vi "Measurement UI.vi"() -> ()   [LabVIEW 2021, in "audio_acMeasurement.lvlib"]
uses:
  audio_acMeasurement.lvlib
panel:
  in  "MeasGraphs":T1(tab)
  out "FreqDomainGraph":cluster{"x0":dbl, "dx":dbl, "magnitude":dbl[]}(graph) caption="AC"
  out "TimeDomainGraph":waveform(dbl)(graph) caption="AC"
  out "Channel":string
  out "Spectrum":dbl[](array[numeric])
  out "df":dbl
  out "f0":dbl
  out "Time domain":dbl[](array[numeric])
  out "dt":dbl
  out "THD+N":dbl
  out "THD":dbl
  out "SNR":dbl
  out "Calculated amplitude":dbl
  out "Calculated frequency":dbl
  out "SFDR":dbl
  out "Dynamic range":dbl
  out "Gain error":dbl
  in  "Analog source resource name":string
  out "MeasTable":string[][](table)
  in  "Channel name":string caption="CHANNEL NAME"
  in  "Channel":u32 caption="CHANNEL"
  in  "Data line":u16 caption="DATA LINE"
  out "Calculated sample rate":u32 caption="SAMPLE RATE" format="%#.6pHz"
  in  "Protocol capture resource name":string caption="RESOURCE NAME"
  in  "Protocol settings":string="Protocol settings"
  in  "Analog source":string="Analog source "
  in  "Full scale range":dbl=3.16 caption="FULL SCALE RANGE" format="%.3pV"
  in  "Measurement settings":string="Measurement settings"
  in  "MeasSettingsOptions":i32(listbox)=-1
  in  "MeasSettings":bool
  in  "Protocol":u16(ring) caption="PROTOCOL" items=["I2S"]
  in  "DSGResourceName":tag caption="RESOURCE NAME"
  in  "Weighting filter":T2(ring) caption="WEIGHTING FILTER"
  in  "Number of words":i32=19200 caption="NUMBER OF WORDS"
  in  "Clock rate":u32=12288000 caption="CLOCK RATE" format="%#.6pHz"
  in  "Band stop":dbl=20000.0 caption="BAND STOP" format="%#_6pHz"
  in  "Band start":dbl=20.0 caption="BAND START" format="%#_6pHz"
  in  "Amplitude":dbl=-1.0 caption="AMPLITUDE" format="%#_6pdB"
  in  "Frequency":dbl=1000.0 caption="FREQUENCY" format="%#_6pHz"
  in  "Sensitivity":dbl=0.34762 caption="SENSITIVITY" format="%.5fFS/Pa"
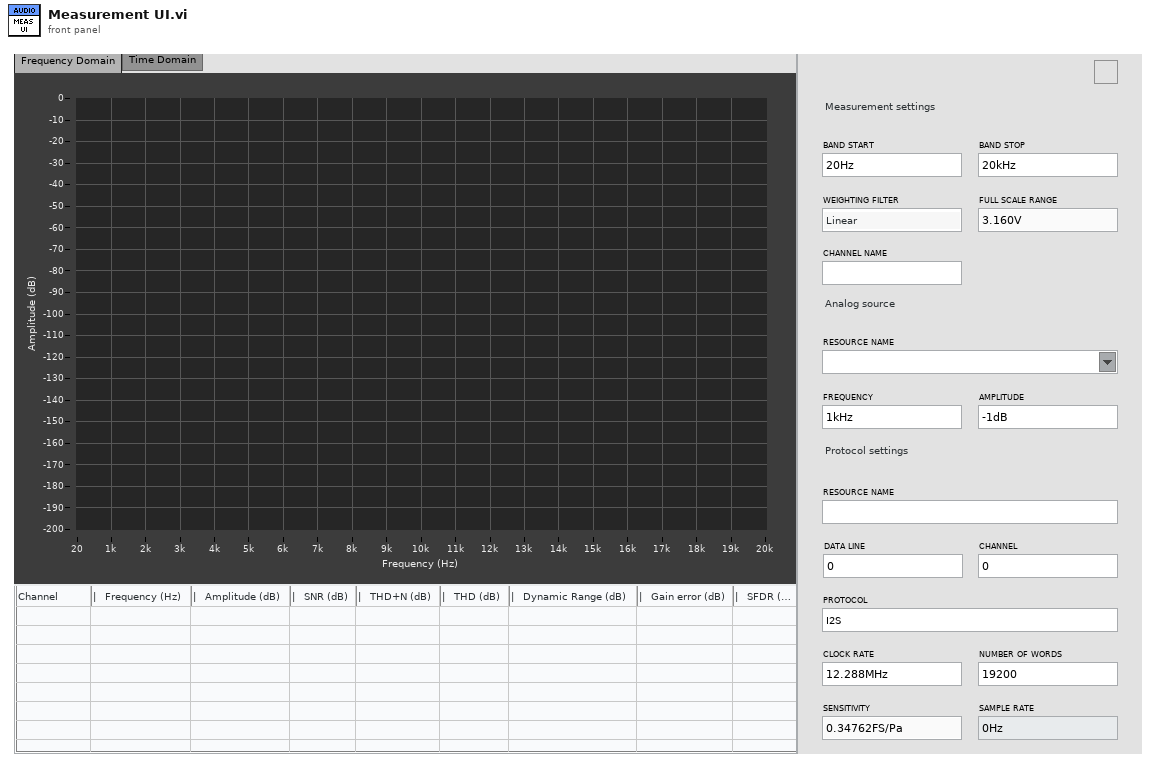
[diagram p1: front panel]
types:
  T1 = enum32{"Frequency Domain", "Time Domain", "Hidden Controls"}
  T2 = enum16{"Linear", "A-Weighting", "B-Weighting", "C-Weighting"}
  T3 = enum16{"open", "replace", "create", "open or create", "replace or create", "replace or create with confirmation"}
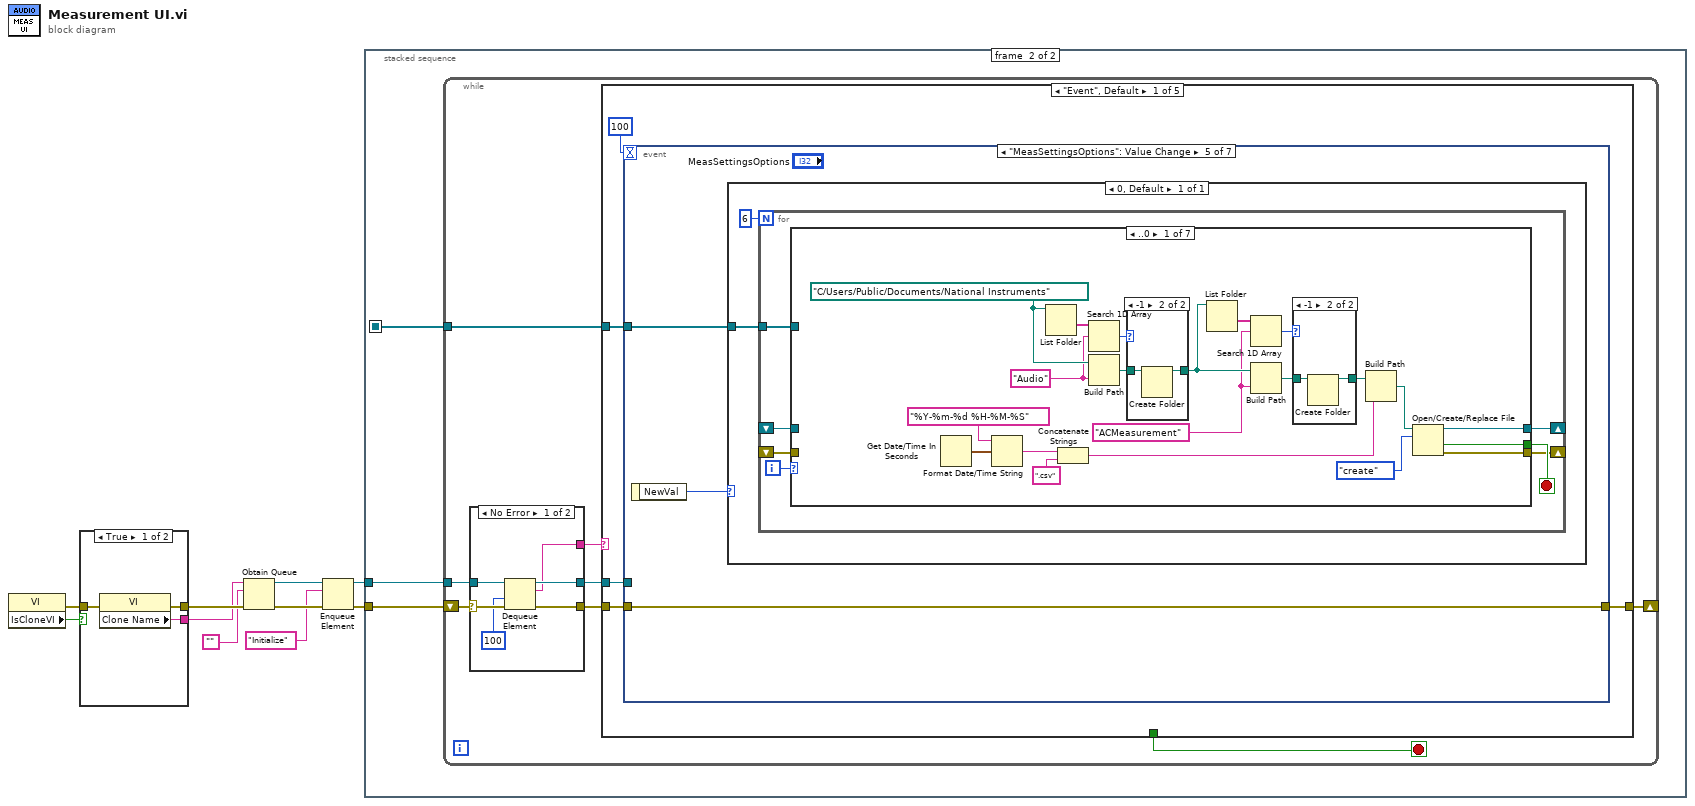
[diagram p0: block diagram]
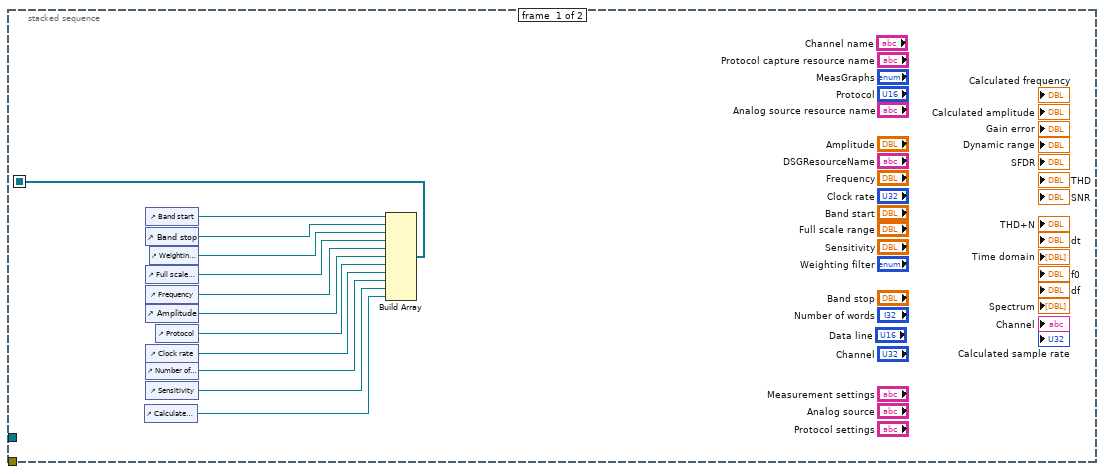
[diagram p2: hidden frame]
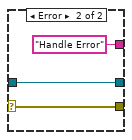
[diagram p3: hidden frame]
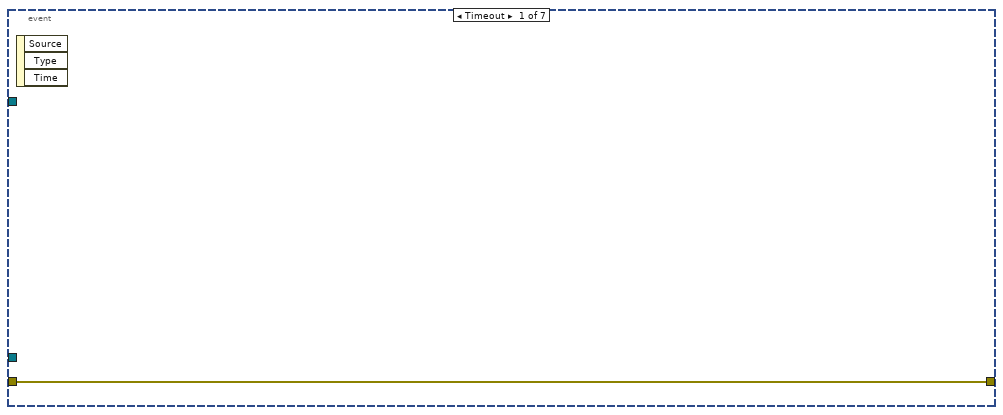
[diagram p4: hidden frame]
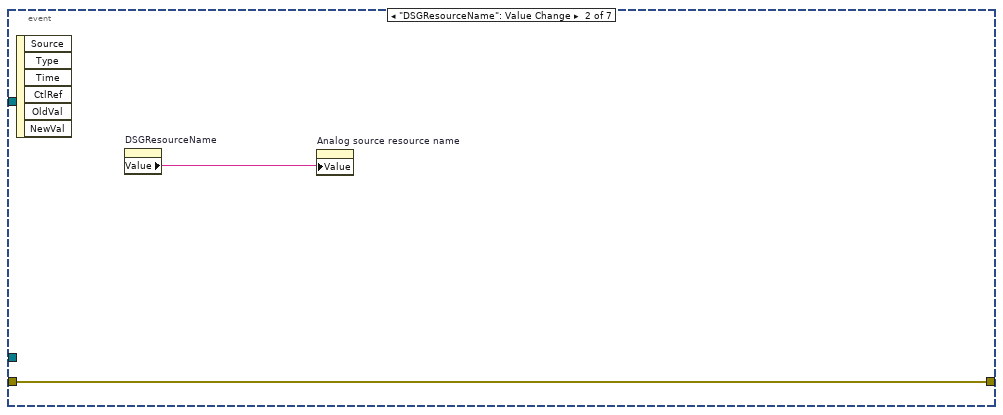
[diagram p5: hidden frame]
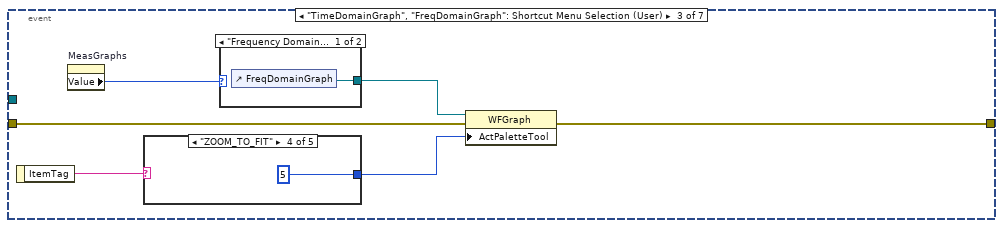
[diagram p6: hidden frame]
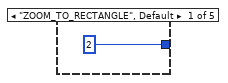
[diagram p7: hidden frame]
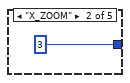
[diagram p8: hidden frame]
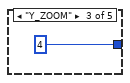
[diagram p9: hidden frame]
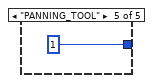
[diagram p10: hidden frame]
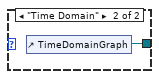
[diagram p11: hidden frame]
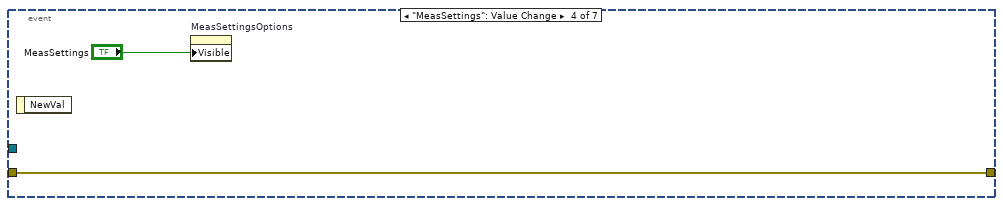
[diagram p12: hidden frame]
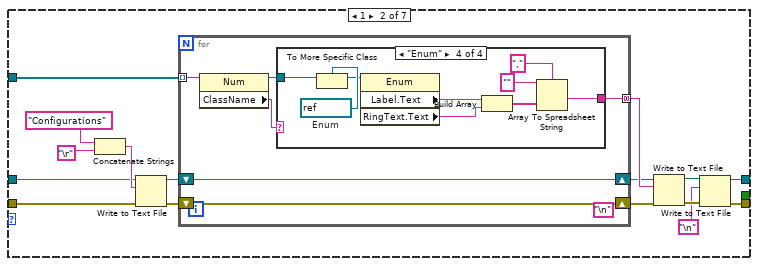
[diagram p15: hidden frame]
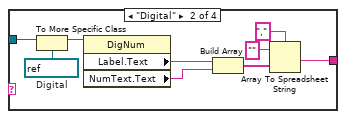
[diagram p17: hidden frame]
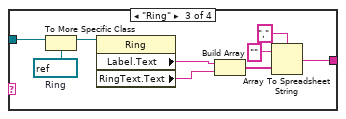
[diagram p18: hidden frame]
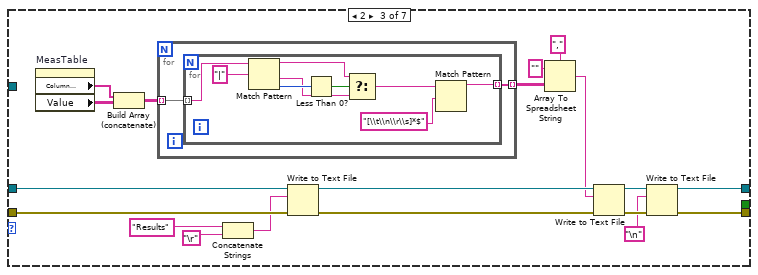
[diagram p19: hidden frame]
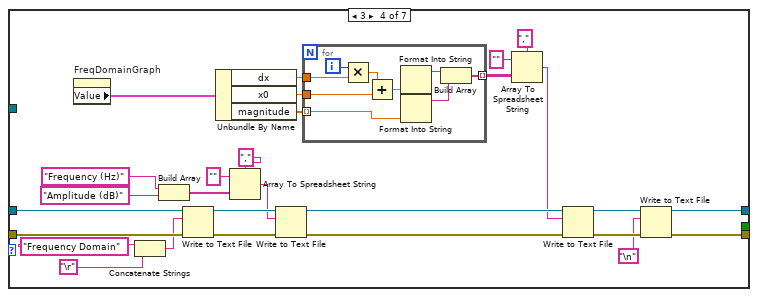
[diagram p20: hidden frame]
diagram:
  n1 = property class="VI"() -> (error out=w1:errorcluster, "IsCloneVI"=w2:bool)  [unwired: 2 in, 1 out]
  n2 = case shown="True" w2 {
    tunnel: [w13 w16] -> w10
    tunnel: [w12 w15] -> w9
    tunnel: w1 -> [w11 w14]
    frame True {
      n3 = property class="VI"(error in=w11) -> (error out=w13:errorcluster, "Clone Name"=w12:string)  [unwired: 1 in, 1 out]
    }
    frame False {
      n4 = property class="VI"(error in=w14) -> (error out=w16:errorcluster, "Name"=w15:string)  [unwired: 1 in, 1 out]
    }
  }
  n5 = Obtain Queue(name (unnamed)=w9, element data type="", error in (no error)=w10) -> (queue out=w6:refnum<queue>, error out=w8:errorcluster)  [unwired: 2 in, 1 out]
  n6 = Enqueue Element(queue=w6, element="Initialize", error in (no error)=w8) -> (queue out=w5:refnum<queue>, error out=w7:errorcluster)  [unwired: 1 in, 1 out]
  n7 = stacked-sequence {
    seq-local: [w25 _] -> [_ w29]
    tunnel: w7 -> [_ w31]
    tunnel: w5 -> [_ w30]
    frame #0 {
      n8 = control-ref of="Calculated sample rate"() -> (w17:refnum<vi>)
      n9 = control-ref of="Band start"() -> (w28:refnum<vi>)
      n10 = control-ref of="Band stop"() -> (w27:refnum<vi>)
      n11 = control-ref of="Full scale range"() -> (w24:refnum<vi>)
      n12 = control-ref of="Frequency"() -> (w21:refnum<vi>)
      n13 = control-ref of="Amplitude"() -> (w20:refnum<vi>)
      n14 = control-ref of="Clock rate"() -> (w23:refnum<vi>)
      n15 = control-ref of="Number of words"() -> (w19:refnum<vi>)
      n16 = control-ref of="Sensitivity"() -> (w18:refnum<vi>)
      n17 = control-ref of="Weighting filter"() -> (w26:refnum<vi>)
      n18 = control-ref of="Protocol"() -> (w22:refnum<vi>)
      n19 = Build Array(w28, w27, w26, w24, w21, w20, w22, w23, w19, w18, w17) -> (w25:refnum<vi>[])
    }
    frame #1 {
      n20 = while {
        shift-right: [w34] -> _
        shift-left: w31 -> [w39]
        tunnel: w30 -> [w37]
        tunnel: w29 -> [w32]
        stop <- w33 stop-if-true
        n21 = case shown="No Error" w39 {
          selector: w39 -> [w45 w48]
          tunnel: [w44 w48] -> w38
          tunnel: w37 -> [w43 w47]
          tunnel: [w42 w47] -> w36
          tunnel: [w41 "Handle Error"] -> w35
          frame No Error {
            n22 = Dequeue Element(queue=w43, timeout in ms (-1)=100, error in (no error)=w45) -> (queue out=w42:refnum<queue>, element=w41:string, error out=w44:errorcluster)  [unwired: 1 out]
          }
          frame Error {
          }
        }
        n23 = case shown="\"Event\", Default" w35 {
          tunnel: w38 -> [w52 w280 w318 w333 w334]
          tunnel: w36 -> [w50 _ _ w331 _]
          tunnel: [w53 w280 w318 w328 w334] -> w34
          tunnel: [_ _ _ TRUE _] -> w33
          tunnel: w32 -> [w49 _ _ _ _]
          frame "Event", Default {
            n24 = event shown="[4] \"MeasSettingsOptions\": Value Change" {
              selector: _ -> [_ _ _ _ _ _ _]
              dyn-events: _ -> [_ _ _ _ _ _ _]
              timeout: 100 -> [_ _ _ _ _ _ _]
              tunnel: [w54 w55 w59 _ w74 w266 w271] -> w53
              tunnel: w52 -> [w54 w55 w58 w70 w74 w266 w272]
              tunnel: w50 -> [_ _ _ _ _ _ w270]
              tunnel: [_ _ _ w70 _ _ _] -> _
              tunnel: w49 -> [_ _ _ _ w72 _ _]
              event Timeout {
                n25 = event-data() -> ()  [unwired: 1 in, 3 out]
              }
              event "DSGResourceName": Value Change {
                n26 = event-data() -> ()  [unwired: 1 in, 6 out]
                n27 = property on="DSGResourceName" class="DAQmxName"() -> ("Value"=w56:string)  [unwired: 2 in, 2 out]
                n28 = property on="Analog source resource name" class="Str"("Value"=w56) -> ()  [unwired: 2 in, 2 out]
              }
              event "TimeDomainGraph", "FreqDomainGraph": Shortcut Menu Selection (User) {
                n29 = event-data() -> ("ItemTag"=w61:string)  [unwired: 1 in]
                n30 = property on="MeasGraphs" class="TabCtl (strict)"() -> ("Value"=w62:T1)  [unwired: 2 in, 2 out]
                n31 = case shown="\"ZOOM_TO_FIT\"" w61 {
                  tunnel: [2 3 4 5 1] -> w57
                  frame "ZOOM_TO_RECTANGLE", Default {
                  }
                  frame "X_ZOOM" {
                  }
                  frame "Y_ZOOM" {
                  }
                  frame "ZOOM_TO_FIT" {
                  }
                  frame "PANNING_TOOL" {
                  }
                }
                n32 = case shown="\"Frequency Domain\", Default" w62 {
                  tunnel: [w68 w69] -> w60
                  frame "Frequency Domain", Default {
                    n33 = control-ref of="FreqDomainGraph"() -> (w68:refnum<vi>)
                  }
                  frame "Time Domain" {
                    n34 = control-ref of="TimeDomainGraph"() -> (w69:refnum<vi>)
                  }
                }
                n35 = property class="WFGraph"(reference=w60, error in=w58, "ActPaletteTool"=w57) -> (error out=w59:errorcluster)  [unwired: 1 out]
              }
              event "MeasSettings": Value Change {
                n36 = event-data() -> ()  [unwired: 1 in, 1 out]
                n37 = property on="MeasSettingsOptions" class="LstBox (strict)"("Visible"="MeasSettings") -> ()  [unwired: 2 in, 2 out]
              }
              event "MeasSettingsOptions": Value Change {
                n38 = event-data() -> ("NewVal"=w73:i32)  [unwired: 1 in]
                n39 = case shown="0, Default" w73 {
                  tunnel: w72 -> [w75]
                  frame 0, Default {
                    n40 = for {
                      N: 6 -> [_]
                      shift-right: [w81] -> _
                      shift-left: _ -> [w80]
                      shift-right: [w79] -> _
                      shift-left: _ -> [w78]
                      tunnel: w75 -> [w77]
                      i -> [w83]
                      stop <- w82 stop-if-true
                      n41 = case shown="..0" w83 {
                        tunnel: [w97 _ _ _ _ _ _] -> w82
                        tunnel: [w103 w123 w167 w194 w235 refnum<file> refnum ("refnum out") w265] -> w81
                        tunnel: w80 -> [_ w120 w178 w217 w236 w263 w265]
                        tunnel: [w96 w122 w166 w192 w234 w261 w264] -> w79
                        tunnel: w78 -> [_ w118 w177 w216 w237 w260 w264]
                        tunnel: w77 -> [_ w121 _ _ _ _ _]
                        frame ..0 {
                          w92 = "ACMeasurement" ("prompt")
                          w99 = "Audio" ("prompt")
                          w102 = path "C:/Users/Public/Documents/National Instruments" ("base path")
                          n42 = Get Date/Time In Seconds() -> (seconds since 1Jan1904=w89:timestamp)
                          n43 = Format Date/Time String(time format string (%c)="%Y-%m-%d %H-%M-%S", seconds (now)=w89) -> (date/time string=w88:string)  [unwired: 1 in]
                          n44 = List Folder(path=w102) -> (folder names=w100:string[])  [unwired: 3 in, 3 out]
                          n45 = Concatenate Strings(w88, ".csv" ("string")) -> (w85:string)
                          n46 = Search 1D Array(1D array=w100, element=w99) -> (index of element=w98:i32)  [unwired: 1 in]
                          n47 = Build Path(base path=w102, name or relative path=w99) -> (appended path=w101:path)
                          n48 = case shown="-1" w98 {
                            tunnel: w101 -> [w108 w110]
                            tunnel: [w108 w109] -> w93
                            frame Default {
                            }
                            frame -1 {
                              n49 = Create Folder(path (use dialog)=w110) -> (created path=w109:path)  [unwired: 2 in, 2 out]
                            }
                          }
                          n50 = List Folder(path=w93) -> (folder names=w95:string[])  [unwired: 3 in, 3 out]
                          n51 = Search 1D Array(1D array=w95, element=w92) -> (index of element=w94:i32)  [unwired: 1 in]
                          n52 = Build Path(base path=w93, name or relative path=w92) -> (appended path=w91:path)
                          n53 = case shown="-1" w94 {
                            tunnel: w91 -> [w105 w107]
                            tunnel: [w105 w106] -> w86
                            frame Default {
                            }
                            frame -1 {
                              n54 = Create Folder(path (use dialog)=w107) -> (created path=w106:path)  [unwired: 2 in, 2 out]
                            }
                          }
                          n55 = Build Path(base path=w86, name or relative path=w85) -> (appended path=w84:path)
                          n56 = Open/Create/Replace File(file path (use dialog)=w84, operation (0:open)=T3."create") -> (refnum out=w103:refnum<file>, cancelled=w97:bool, error out=w96:errorcluster)  [unwired: 4 in]
                        }
                        frame 1 {
                          (unwired) "\n"
                          n57 = Concatenate Strings("Configurations" ("format string"), "\r") -> (w124:string)
                          n58 = Write to Text File(file (use dialog)=w120, text=w124, error in=w118) -> (refnum out=w117:refnum<file>, error out=w119:errorcluster)  [unwired: 1 in, 1 out]
                          n59 = for {
                            tunnel: w121 -> [w128] mode=indexing
                            shift-right: [w132] -> w115
                            shift-left: w117 -> [w132]
                            shift-right: [w131] -> w114
                            shift-left: w119 -> [w131]
                            tunnel: [w130] -> w116 mode=concatenating
                            n60 = property class="Num"(reference=w128) -> (reference out=w129:refnum<vi>, "ClassName"=w127:string)  [unwired: 1 in, 1 out]
                            n61 = case shown="\"Enum\"" w127 {
                              tunnel: [_ w136 w146 w155] -> w130
                              tunnel: w129 -> [_ w134 w144 w159]
                              frame Default {
                              }
                              frame "Digital" {
                                w133 = refnum<vi> refnum  # Digital
                                n62 = To More Specific Class(target class=w133, reference=w134) -> (specific class reference=w135:refnum<vi>)  [unwired: 1 in, 1 out]
                                n63 = property class="DigNum"(reference=w135) -> ("Label.Text"=w141:string, "NumText.Text"=w140:string)  [unwired: 1 in, 2 out]
                                n64 = Build Array(w141, w140) -> (w137:string[])
                                n65 = Array To Spreadsheet String(delimiter (Tab)=",", array=w137, 3:"" ("format string")) -> (spreadsheet string=w136:string)
                              }
                              frame "Ring" {
                                w143 = refnum<vi> refnum  # Ring
                                n66 = To More Specific Class(target class=w143, reference=w144) -> (specific class reference=w145:refnum<vi>)  [unwired: 1 in, 1 out]
                                n67 = property class="Ring"(reference=w145) -> ("Label.Text"=w142:string, "RingText.Text"=w150:string)  [unwired: 1 in, 2 out]
                                n68 = Build Array(w142, w150) -> (w147:string[])
                                n69 = Array To Spreadsheet String(delimiter (Tab)=",", array=w147, 3:"" ("format string")) -> (spreadsheet string=w146:string)
                              }
                              frame "Enum" {
                                w158 = refnum<vi> refnum  # Enum
                                n70 = To More Specific Class(target class=w158, reference=w159) -> (specific class reference=w154:refnum<vi>)  [unwired: 1 in, 1 out]
                                n71 = property class="Enum"(reference=w154) -> ("Label.Text"=w153:string, "RingText.Text"=w152:string)  [unwired: 1 in, 2 out]
                                n72 = Build Array(w153, w152) -> (w151:string[])
                                n73 = Array To Spreadsheet String(delimiter (Tab)=",", array=w151, 3:"" ("format string")) -> (spreadsheet string=w155:string)
                              }
                            }
                          }
                          n74 = Write to Text File(file (use dialog)=w115, text=w116, error in=w114) -> (refnum out=w113:refnum<file>, error out=w112:errorcluster)  [unwired: 1 in, 1 out]
                          n75 = Write to Text File(file (use dialog)=w113, text="\n", error in=w112) -> (refnum out=w123:refnum<file>, error out=w122:errorcluster)  [unwired: 1 in, 1 out]
                        }
                        frame 2 {
                          n76 = property on="MeasTable" class="Tbl (strict)"() -> ("Column Headers[]"=w161:string[], "Value"=w160:string[][])  [unwired: 2 in, 2 out]
                          n77 = Build Array (concatenate)(w161, w160) -> (w175:string[][])
                          n78 = for {
                            tunnel: w175 -> [w180] mode=indexing
                            tunnel: [w179] -> w174 mode=indexing
                            n79 = for {
                              tunnel: w180 -> [w182] mode=indexing
                              tunnel: [w181] -> w179 mode=indexing
                              n80 = Match Pattern(string=w182, regular expression="|") -> (before substring=w186:string, after substring=w185:string, offset past match=w188:i32)  [unwired: 1 in, 1 out]
                              n81 = Less Than 0?(x=w188) -> (x < 0?=w187:bool)
                              n82 = Select(t=w186, s=w187, f=w185) -> (s? t:f=w184:string)
                              n83 = Match Pattern(string=w184, regular expression="[\\t\\n\\r\\s]*$") -> (before substring=w181:string)  [unwired: 1 in, 3 out]
                            }
                          }
                          n84 = Concatenate Strings("Results" ("element"), "\r") -> (w162:string)
                          n85 = Write to Text File(file (use dialog)=w178, text=w162, error in=w177) -> (refnum out=w176:refnum<file>, error out=w170:errorcluster)  [unwired: 1 in, 1 out]
                          n86 = Array To Spreadsheet String(delimiter (Tab)=",", array=w174, 3:"" ("format string")) -> (spreadsheet string=w171:string)
                          n87 = Write to Text File(file (use dialog)=w176, text=w171, error in=w170) -> (refnum out=w169:refnum<file>, error out=w168:errorcluster)  [unwired: 1 in, 1 out]
                          n88 = Write to Text File(file (use dialog)=w169, text="\n", error in=w168) -> (refnum out=w167:refnum<file>, error out=w166:errorcluster)  [unwired: 1 in, 1 out]
                        }
                        frame 3 {
                          n89 = property on="FreqDomainGraph" class="WFGraph (strict)"() -> ("Value"=w197:cluster{"x0":dbl, "dx":dbl, "magnitude":dbl[]})  [unwired: 2 in, 2 out]
                          n90 = Concatenate Strings("Frequency Domain" ("string"), "\r") -> (w214:string)
                          n91 = Build Array("Frequency (Hz)", "Amplitude (dB)") -> (w213:string[])
                          n92 = Write to Text File(file (use dialog)=w217, text=w214, error in=w216) -> (refnum out=w210:refnum<file>, error out=w209:errorcluster)  [unwired: 1 in, 1 out]
                          n93 = Unbundle By Name(w197) -> ("dx"=w201:dbl, "x0"=w202:dbl, "magnitude"=w200:dbl[])
                          n94 = Array To Spreadsheet String(delimiter (Tab)=",", array=w213, 3:"" ("format string")) -> (spreadsheet string=w208:string)
                          n95 = Write to Text File(file (use dialog)=w210, text=w208, error in=w209) -> (refnum out=w207:refnum<file>, error out=w206:errorcluster)  [unwired: 1 in, 1 out]
                          n96 = for {
                            tunnel: w200 -> [w221] mode=indexing
                            tunnel: w201 -> [w225]
                            tunnel: w202 -> [w223]
                            tunnel: [w218] -> w203 mode=indexing
                            i -> [w226]
                            n97 = Multiply(x=w226, y=w225) -> (x*y=w224:dbl)
                            n98 = Add(x=w224, y=w223) -> (x+y=w222:dbl)
                            n99 = Format Into String(w222) -> (resulting string=w219:string)  [unwired: 3 in, 1 out]
                            n100 = Format Into String(w221) -> (resulting string=w220:string)  [unwired: 3 in, 1 out]
                            n101 = Build Array(w219, w220) -> (w218:string[])
                          }
                          n102 = Array To Spreadsheet String(delimiter (Tab)=",", array=w203, 3:"" ("format string")) -> (spreadsheet string=w199:string)
                          n103 = Write to Text File(file (use dialog)=w207, text=w199, error in=w206) -> (refnum out=w196:refnum<file>, error out=w195:errorcluster)  [unwired: 1 in, 1 out]
                          n104 = Write to Text File(file (use dialog)=w196, text="\n", error in=w195) -> (refnum out=w194:refnum<file>, error out=w192:errorcluster)  [unwired: 1 in, 1 out]
                        }
                        frame 4 {
                          n105 = property on="TimeDomainGraph" class="WFGraph (strict)"() -> ("Value"=w233:waveform(dbl))  [unwired: 2 in, 2 out]
                          n106 = Concatenate Strings("Time Domain" ("string"), "\r") -> (w249:string)
                          n107 = Write to Text File(file (use dialog)=w236, text=w249, error in=w237) -> (refnum out=w246:refnum<file>, error out=w245:errorcluster)  [unwired: 1 in, 1 out]
                          n108 = Build Array("Time (s)", "Amplitude (V)") -> (w248:string[])
                          n109 = Unbundle By Name(w233) -> ("dt"=w231:dbl, "Y"=w232:dbl[])
                          n110 = Array To Spreadsheet String(delimiter (Tab)=",", array=w248, 3:"" ("format string")) -> (spreadsheet string=w244:string)
                          n111 = Write to Text File(file (use dialog)=w246, text=w244, error in=w245) -> (refnum out=w243:refnum<file>, error out=w242:errorcluster)  [unwired: 1 in, 1 out]
                          n112 = for {
                            tunnel: [w255] -> w239 mode=indexing
                            tunnel: w232 -> [w254] mode=indexing
                            tunnel: w231 -> [w252]
                            i -> [w253]
                            n113 = Multiply(x=w252, y=w253) -> (x*y=w251:dbl)
                            n114 = Format Into String(w251) -> (resulting string=w256:string)  [unwired: 3 in, 1 out]
                            n115 = Format Into String(w254) -> (resulting string=w257:string)  [unwired: 3 in, 1 out]
                            n116 = Build Array(w256, w257) -> (w255:string[])
                          }
                          n117 = Array To Spreadsheet String(delimiter (Tab)=",", array=w239, 3:"" ("format string")) -> (spreadsheet string=w238:string)
                          n118 = Write to Text File(file (use dialog)=w243, text=w238, error in=w242) -> (refnum out=w235:refnum<file>, error out=w234:errorcluster)  [unwired: 1 in, 1 out]
                        }
                        frame 5 {
                          w258 = FALSE ("Visible")
                          n119 = Close File(refnum=w263, error in=w260) -> (error out=w261:errorcluster)  [unwired: 1 out]
                          n120 = property on="MeasSettingsOptions" class="LstBox (strict)"("Visible"=w258, "Value"=-1 ("MeasSettingsOptions")) -> ()  [unwired: 2 in, 2 out]
                          n121 = property on="MeasSettings" class="Bool (strict)"("Value"=w258) -> ()  [unwired: 2 in, 2 out]
                        }
                        frame Default {
                        }
                      }
                    }
                  }
                }
              }
              event Mouse Down {
                w267 = FALSE ("Visible")
                n122 = event-data() -> ()  [unwired: 1 in, 1 out]
                n123 = property on="MeasSettingsOptions" class="LstBox (strict)"("Visible"=w267, "Value"=-1 ("MeasSettingsOptions")) -> ()  [unwired: 2 in, 2 out]
                n124 = property on="MeasSettings" class="Bool (strict)"("Value"=w267) -> ()  [unwired: 2 in, 2 out]
              }
              event Panel Close? {
                n125 = event-data() -> ()  [unwired: 1 in, 4 out]
                n126 = Enqueue Element(queue=w270, element="Exit", error in (no error)=w272) -> (error out=w271:errorcluster)  [unwired: 1 in, 2 out]
                n127 = event-data("Discard?"=TRUE) -> ()  [unwired: 1 in, 1 out]
              }
            }
          }
          frame "Initialize" {
            w278 = string[] ["Export data"] ("Item Names")
            w274 = "<Select Device>"
            n128 = for {
              N: 2 -> [_]
              i -> [w283]
              n129 = case shown="0, Default" w283 {
                tunnel: [w286 w287] -> w284
                frame 0, Default {
                  n130 = control-ref of="FreqDomainGraph"() -> (w286:refnum<vi>)
                }
                frame 1 {
                  n131 = control-ref of="TimeDomainGraph"() -> (w287:refnum<vi>)
                }
              }
              n132 = property class="WFGraph"(reference=w284, "ActPaletteTool"=2 ("Palette:Active Tool")) -> ()  [unwired: 1 in, 2 out]
            }
            n133 = property on="DSGResourceName" class="DAQmxName"("Value"=w274) -> ()  [unwired: 2 in, 2 out]
            n134 = property on="Protocol capture resource name" class="Str"("Value"=w274) -> ()  [unwired: 2 in, 2 out]
            n135 = property on="MeasSettingsOptions" class="LstBox (strict)"("Item Names"=w278, "Value"=-1 ("MeasSettingsOptions"), "Visible"=FALSE, "Disabled Items"=i32[] []) -> ()  [unwired: 2 in, 2 out]
            n136 = for {
              tunnel: w278 -> [_] mode=indexing
              i -> [w282]
              n137 = property on="MeasSettingsOptions" class="LstBox (strict)"("Active Row"=w282, "Cell Height"=30 ("Active Row:Cell Height")) -> ()  [unwired: 2 in, 2 out]
            }
          }
          frame "Post UI Update" {
            w300 = "|   " ("initial string")
            # "This case will be triggered, after framework updates the User interface with result values."
            n138 = local read "Time domain"() -> (w317:dbl[])
            n139 = local read "Spectrum"() -> (w291:dbl[])
            n140 = local read "df"() -> (w293:dbl)
            n141 = local read "dt"() -> (w316:dbl)
            n142 = local read "f0"() -> (w290:dbl)
            n143 = local read "Calculated frequency"() -> (w303:dbl)
            n144 = local read "Calculated amplitude"() -> (w302:dbl)
            n145 = local read "Dynamic range"() -> (w312:dbl)
            n146 = Bundle By Name("Y"=w317, "dt"=w316) -> (→"TimeDomainGraph":waveform(dbl))  [unwired: 1 in]
            n147 = Bundle(cluster=cluster{"x0":dbl, "dx":dbl, "magnitude":dbl[]} {"x0"=0.0, "dx"=0.0, "magnitude"=[]} ("FreqDomainGraph"), "x0"=w290, "dx"=w293, "magnitude"=w291) -> (→"FreqDomainGraph":cluster{"x0":dbl, "dx":dbl, "magnitude":dbl[]})
            n148 = local read "THD+N"() -> (w313:dbl)
            n149 = local read "Gain error"() -> (w299:dbl)
            n150 = local read "THD"() -> (w314:dbl)
            n151 = local read "SNR"() -> (w301:dbl)
            n152 = local read "SFDR"() -> (w298:dbl)
            n153 = Build Array(w303, w302) -> (w309:dbl[])
            n154 = Build Array(w301, w313, w314, w312) -> (w308:dbl[])
            n155 = for {
              tunnel: w309 -> [w323] mode=indexing
              tunnel: w300 -> [w324]
              tunnel: "%.3f" ("initial string") -> [w325]
              tunnel: [w326] -> w307 mode=indexing
              n156 = Format Into String(format string=w325, initial string=w324, w323) -> (resulting string=w326:string)  [unwired: 1 in, 1 out]
            }
            n157 = for {
              tunnel: w308 -> [w319] mode=indexing
              tunnel: w300 -> [w320]
              tunnel: "%5.1f" ("initial string") -> [w321]
              tunnel: [w322] -> w306 mode=indexing
              n158 = Format Into String(format string=w321, initial string=w320, w319) -> (resulting string=w322:string)  [unwired: 1 in, 1 out]
            }
            n159 = Format Into String(format string="%5.1f" ("initial string"), initial string=w300, w298) -> (resulting string=w296:string)  [unwired: 1 in, 1 out]
            n160 = Format Into String(format string="%5.3f" ("initial string"), initial string=w300, w299) -> (resulting string=w297:string)  [unwired: 1 in, 1 out]
            n161 = local read "Channel"() -> (w288:string)
            n162 = Build Array (concatenate)(w288, w307, w306, w297, w296) -> (w305:string[])
            n163 = Build Array(w305) -> (→"MeasTable":string[][])
          }
          frame "Exit" {
            # "This case is triggered to close the User Interface from framework"
            n164 = Flush Queue(queue=w331, error in (no error)=w333) -> (queue out=w330:refnum<queue>, error out=w329:errorcluster)  [unwired: 1 out]
            n165 = Release Queue(queue=w330, force destroy? (F)=TRUE, error in (no error)=w329) -> (error out=w328:errorcluster)  [unwired: 2 out]
          }
          frame "Handle Error" {
          }
        }
      }
    }
  }
